vi "New RegReadExt Command.vi"(0 "RFFE RegReadExt Command in":refnum<class "RFFE RegReadExt Command.lvclass">, 5 "Slave Address":T2=12 format="%02x", 7 "Register Address":T1 format="%02x", 9 "Byte Count":i32=1, 11 "error in (no error)":errorcluster) -> (4 "RFFE RegReadExt Command out":refnum<class "RFFE RegReadExt Command.lvclass">, 15 "error out":errorcluster)   [LabVIEW 2018, in "MIPI RFFE API.lvlib" / "RFFE RegReadExt Command.lvclass"]
uses:
  RFFE RegReadExt Command.lvclass
  C:/Users/semoore/Projects/mipi-rffe-labview-oop/Extended Command/RFFE Extended Command.lvclass
  Slave Address.ctl
  Register Address.ctl
  Register Data.ctl
  RFFE RegReadExt Command.lvclass/RFFE RegReadExt Command.ctl
  Extended Command/RFFE Extended Command.lvclass
  MIPI RFFE API.lvlib
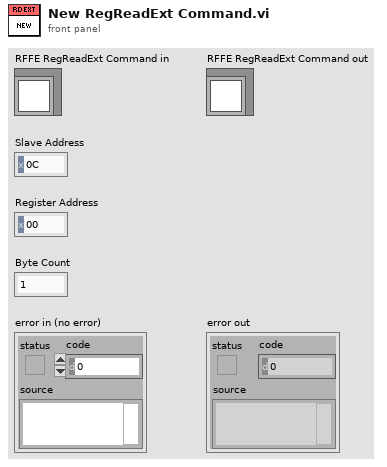
[diagram p1: front panel]
types:
  T1 = typedef "MIPI RFFE API.lvlib/Register Address.ctl" = u16
  T2 = typedef "MIPI RFFE API.lvlib/Slave Address.ctl" = u8
  T3 = typedef "MIPI RFFE API.lvlib/Register Data.ctl" = u8
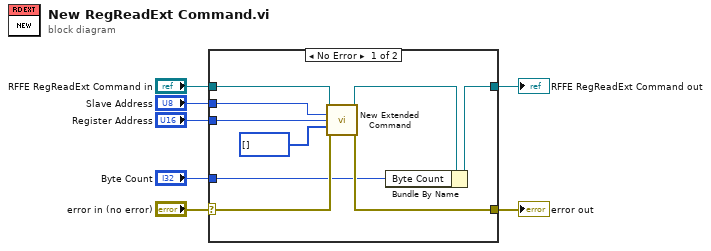
[diagram p0: block diagram]
diagram:
  n1 = case shown="No Error" "error in (no error)" {
    selector: "error in (no error)" -> [w15 w18]
    tunnel: [w14 w18] -> w6
    tunnel: [w9 w17] -> w4
    tunnel: "RFFE RegReadExt Command in" -> [w16 w17]
    tunnel: "Register Address" -> [w13 _]
    tunnel: "Slave Address" -> [w12 _]
    tunnel: "Byte Count" -> [w8 _]
    frame No Error {
      n2 = call "New Extended Command.vi"("RFFE Extended Command in"=w16, "Slave Address"=w12, "Register Address"=w13, "Register Data"=T3[] [], "error in (no error)"=w15) -> ("RFFE Extended Command out"=w10:refnum<class "RFFE RegReadExt Command.lvclass">, "error out"=w14:errorcluster)  [unwired: 9 in]
      n3 = Bundle By Name(cluster=w10, "Byte Count"=w8) -> (w9:refnum<class "RFFE RegReadExt Command.lvclass">)
    }
    frame Error {
    }
  }
  "error out" <- w6
  "RFFE RegReadExt Command out" <- w4
